vi "SSIM - Mean Square Error.vi"(8 "error in":errorcluster, 9 "MSE Map":T1, 10 "Reference Image":T1, 11 "Test Image":T1) -> (0 "error out":errorcluster, 1 "MSE Map Out":T1, 3 "Mean Square Error":dbl)   [LabVIEW 2014]
uses:
  <vilib>/vision/Image Controls.llb/IMAQ Image.ctl
  <vilib>/vision/NI_Vision_Development_Module.lvlib
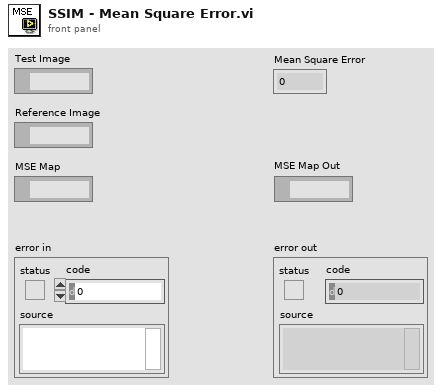
[diagram p1: front panel]
types:
  T1 = typedef "IMAQ Image.ctl" = refnum<image>
  T2 = typedef "Image Type" = u32
  T3 = cluster{"histogram":u32[], "Minimal Value":sgl, "Maximal Value":sgl, "Starting Value":sgl, "Interval Width":sgl, "Mean Value":sgl, "Standard  Variation":sgl, "Area (pixels)":i32}
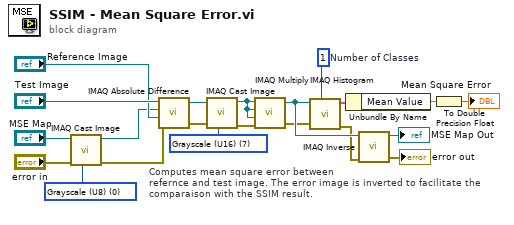
[diagram p0: block diagram]
diagram:
  w11 = T2 0 items=["Grayscale (U8)", "Grayscale (I16)", "Grayscale (SGL)", "Complex (CSG)", "RGB (U32)", "HSL (U32)", "RGB (U64)", "Grayscale (U16)"] ("Image Type")
  w17 = 1  # Number of Classes
  w18 = T2 7 items=["Grayscale (U8)", "Grayscale (I16)", "Grayscale (SGL)", "Complex (CSG)", "RGB (U32)", "HSL (U32)", "RGB (U64)", "Grayscale (U16)"] ("Image Type")
  # "Computes mean square error between\nrefernce and test image. The error image is inverted to facilitate the comparaison with the SSIM result."
  n1 = call "IMAQ Cast Image"("Image Type"=w11, "error in (no error)"="error in", "Image Src"="MSE Map") -> ("error out"=w1:errorcluster, "Image Dst Out"=w9:T1)  [unwired: 3 in, 4 out]
  n2 = call "IMAQ Absolute Difference"("Image Src A"="Test Image", "Image Dst"=w9, "Image Src B"="Reference Image", "error in (no error)"=w1) -> ("Image Dst Out"=w19:T1, "error out"=w7:errorcluster)  [unwired: 1 in, 2 out]
  n3 = call "IMAQ Cast Image"("Image Type"=w18, "error in (no error)"=w7, "Image Src"=w19) -> ("error out"=w6:errorcluster, "Image Dst Out"=w12:T1)  [unwired: 3 in, 4 out]
  n4 = call "IMAQ Multiply"("Image Src A"=w12, "Image Dst"=w12, "Image Src B"=w12, "error in (no error)"=w6) -> ("Image Dst Out"=w16:T1, "error out"=w5:errorcluster)  [unwired: 1 in, 2 out]
  n5 = call "IMAQ Histogram"("Number of Classes"=w17, "error in (no error)"=w5, "Image"=w16) -> ("error out"=w8:errorcluster, "Histogram Report"=w14:T3)  [unwired: 2 in, 5 out]
  n6 = Unbundle By Name(w14) -> ("Mean Value"=w13:sgl)
  n7 = call "IMAQ Inverse"("error in (no error)"=w8, "Image Src"=w16) -> ("error out"=→"error out":errorcluster, "Image Dst Out"=→"MSE Map Out":T1)  [unwired: 2 in, 6 out]
  n8 = To Double Precision Float(number=w13) -> (double precision float=→"Mean Square Error":dbl)
